vi "Load Profile (uSMC).vi"(8 "error in":errorcluster, 9 "axis":i32, 10 "Path":path, 11 "Visa array in":refnum<visa-resource-name>[](array[refnum])) -> (0 "error out":errorcluster, 2 "Loaded":bool, 3 "Visa array out":refnum<visa-resource-name>[](array[refnum]))   [LabVIEW 2010, in "SignalWriterMH110203USBStepperMotor.lvclass"]
uses:
  SignalWriterMH110203USBStepperMotor.lvclass
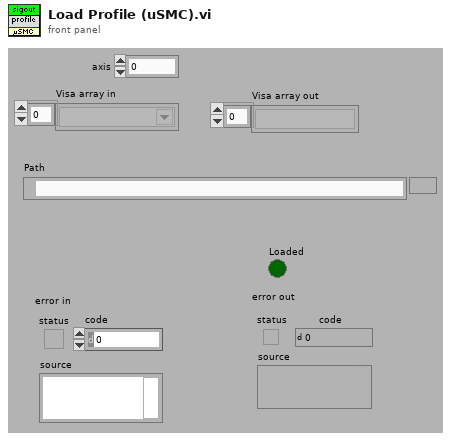
[diagram p1: front panel]
types:
  T1 = enum16{"open", "open or create", "create or replace", "create", "open (read only)"}
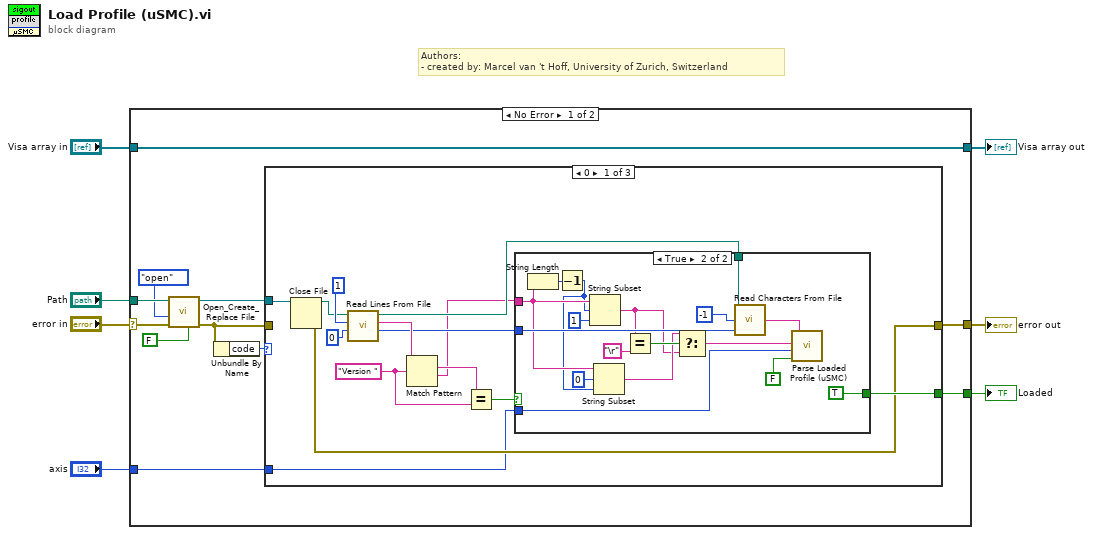
[diagram p0: block diagram]
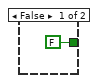
[diagram p2: hidden frame]
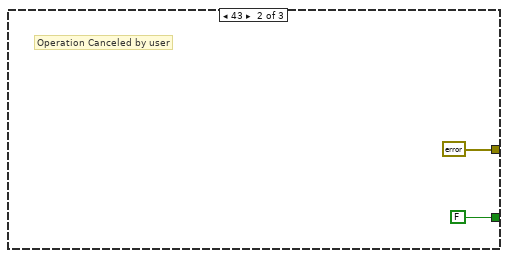
[diagram p3: hidden frame]
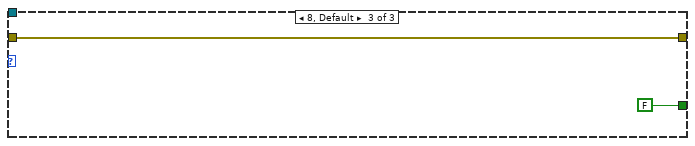
[diagram p4: hidden frame]
diagram:
  # "Authors: \n- created by: Marcel van 't Hoff, University of Zurich, Switzerland"
  n1 = case shown="No Error" "error in" {
    selector: "error in" -> [w10 w56]
    tunnel: "Path" -> [w17 _]
    tunnel: [w14 w56] -> w6
    tunnel: [w13 _] -> w5
    tunnel: "axis" -> [w8 _]
    tunnel: [w9 w55] -> w2
    tunnel: "Visa array in" -> [w9 w55]
    frame No Error {
      n2 = call <vilib>:"Open_Create_Replace File.vi"("advisory dialog? (display:T)"=FALSE, "error in (no error)"=w10, "function (open:0)"=T1."open", "file path"=w17) -> ("error out"=w12:errorcluster, "refnum"=w11:refnum<file>)  [unwired: 4 in, 2 out]
      n3 = Unbundle By Name(w12) -> ("code"=w18:i32)
      n4 = case shown="0" w18 {
        tunnel: w12 -> [_ _ w54]
        tunnel: [w21 errorcluster {"status"=FALSE, "code"=0, "source"=""} ("error out") w54] -> w14
        tunnel: [w23 FALSE FALSE] -> w13
        tunnel: w11 -> [w22 _ _]
        tunnel: w8 -> [w19 _ _]
        frame 0 {
          w29 = "Version " ("regular expression")
          n5 = Close File(refnum=w22) -> (path=w20:path, error out=w21:errorcluster)  [unwired: 1 in]
          n6 = call <vilib>:"Read Lines From File.vi"("file path (dialog if empty)"=w20, "number of lines (all:-1)"=1 ("number of characters (all:-1)"), "start of read offset (chars.:0)"=0) -> ("new file path (Not A Path if cancelled)"=w26:path, "line string"=w30:string, "mark after read (chars.)"=w27:i32)  [unwired: 3 in, 1 out]
          n7 = Match Pattern(string=w30, regular expression=w29) -> (match substring=w28:string, after substring=w25:string)  [unwired: 1 in, 2 out]
          n8 = Equal?(x=w28, y=w29) -> (x = y?=w24:bool)
          n9 = case shown="True" w24 {
            tunnel: w27 -> [_ w49]
            tunnel: w26 -> [_ w48]
            tunnel: w25 -> [_ w47]
            tunnel: [FALSE TRUE] -> w23
            tunnel: w19 -> [_ w34]
            frame False {
            }
            frame True {
              n10 = String Length(string=w47) -> (length=w46:i32)
              n11 = Decrement(x=w46) -> (x-1=w43:i32)
              n12 = String Subset(string=w47, offset (0)=w43, length (rest)=1 ("length (rest)")) -> (substring=w39:string)
              n13 = String Subset(string=w47, offset (0)=0, length (rest)=w43) -> (substring=w40:string)
              n14 = Equal?(x=w39, y="\r") -> (x = y?=w41:bool)
              n15 = Select(t=w40, s=w41, f=w39) -> (s? t:f=w36:string)
              n16 = call <vilib>:"Read Characters From File.vi"("file path (dialog if empty)"=w48, "number of characters (all:-1)"=-1, "start of read offset (chars.:0)"=w49) -> ("character string"=w37:string)  [unwired: 3 in, 3 out]
              n17 = call "Parse Loaded Profile (uSMC).vi"("replace(false)/insert(true)"=FALSE, "SMindex"=w34, "Version"=w36, "data string"=w37) -> ()  [unwired: 2 in]
            }
          }
        }
        frame 43 {
          # "Operation Canceled by user"
        }
        frame 8, Default {
        }
      }
    }
    frame Error {
    }
  }
  "error out" <- w6
  "Loaded" <- w5
  "Visa array out" <- w2
